vi "parse and execute command.vi"(8 "Python Command":string="scan(0,0,64,64)") -> (1 "Python Return String":string="unknown command:scan\r\n", 2 "exit":bool, 3 "command error":errorcluster)   [LabVIEW 2014]
panel:
  out "Command Folder":path
  out "error out":errorcluster={"status"=TRUE, "code"=7, "source"="Open VI Reference in parse and execute command.vi<APPEND>\nVI Path: <b>D:\\Scripts\\VIs\\SLLServer\\NanonisCommand\\scan.vi</b>"}
  in  "VI Refnum":refnum<vi>
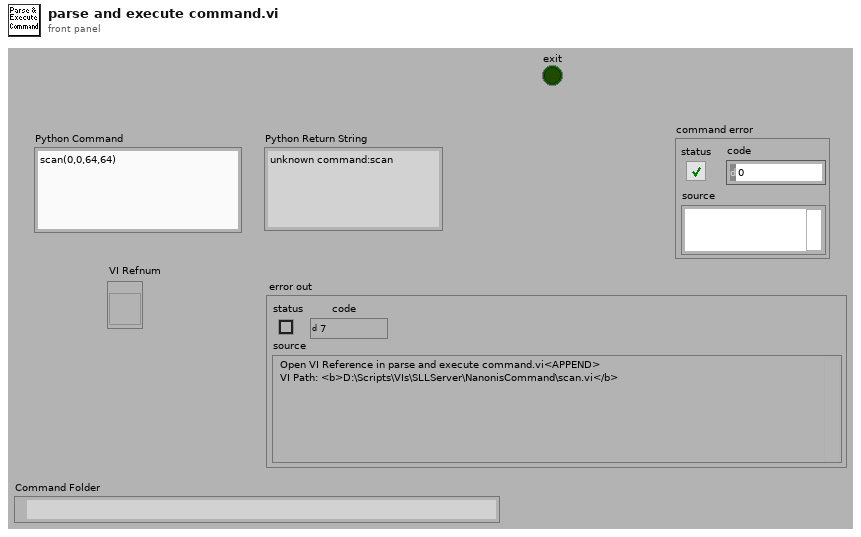
[diagram p1: front panel]
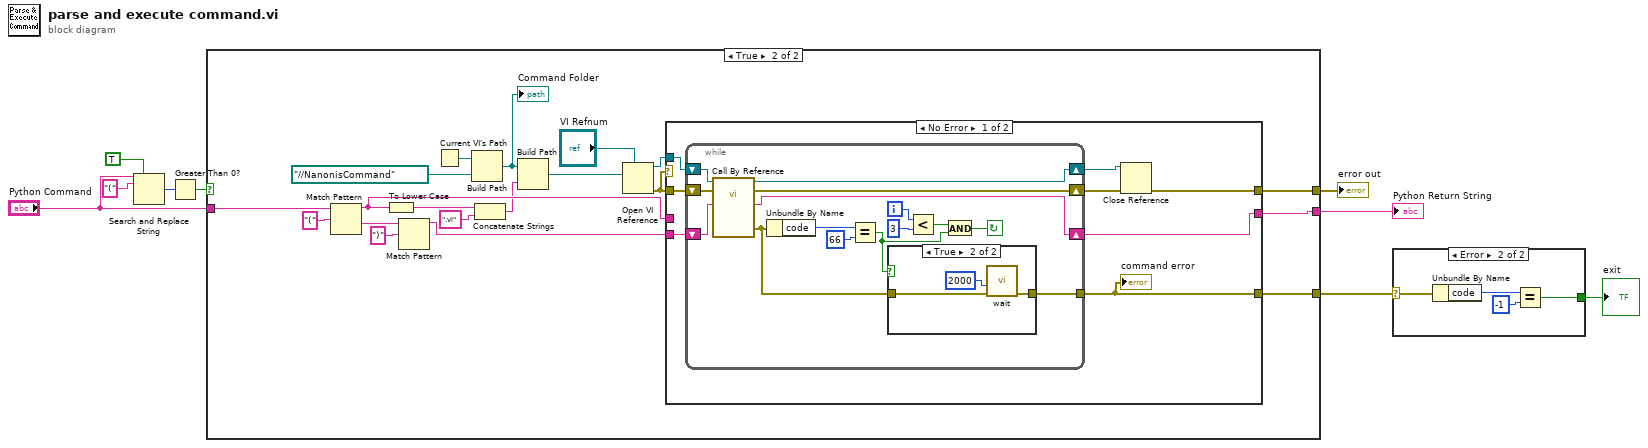
[diagram p0: block diagram]
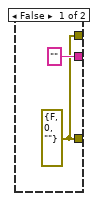
[diagram p2: hidden frame]
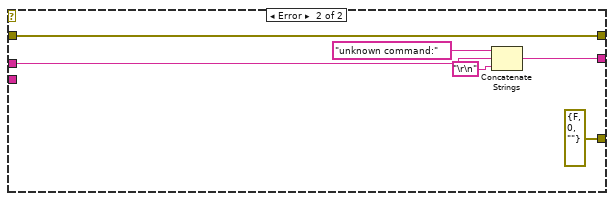
[diagram p4: hidden frame]
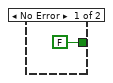
[diagram p5: hidden frame]
diagram:
  n1 = Search and Replace String(replace all?=TRUE ("replace all? (F)"), input string="Python Command", search string="(") -> (number of replacements=w1:i32)  [unwired: 5 in, 3 out]
  n2 = Greater Than 0?(x=w1) -> (x > 0?=w2:bool)
  n3 = case shown="True" w2 {
    tunnel: "Python Command" -> [_ w30]
    tunnel: ["" ("Output") w23] -> w9
    tunnel: [w10 w16] -> w7
    tunnel: [w10 w15] -> w6
    frame False {
      w10 = errorcluster {"status"=FALSE, "code"=0, "source"=""} ("error out")
    }
    frame True {
      n4 = Match Pattern(string=w30, regular expression="(") -> (before substring=w20:string, after substring=w27:string)  [unwired: 1 in, 2 out]
      n5 = To Lower Case(string=w20) -> (all lower case string=w17:string)
      n6 = Match Pattern(string=w27, regular expression=")") -> (before substring=w24:string)  [unwired: 1 in, 3 out]
      n7 = Current VI's Path() -> (path=w13:path)
      n8 = Build Path(base path=w13, name or relative path=path "../../NanonisCommand") -> (appended path=w12:path)
      "Command Folder" <- w12
      n9 = Concatenate Strings(w17, ".vi" ("regular expression")) -> (w18:string)
      n10 = Build Path(base path=w12, name or relative path=w18) -> (appended path=w19:path)
      n11 = Open VI Reference(type specifier VI Refnum (for type only)="VI Refnum", vi path=w19) -> (vi reference=w25:refnum<vi>, error out=w21:errorcluster)  [unwired: 4 in]
      n12 = case shown="No Error" w21 {
        tunnel: w25 -> [w38 _]
        tunnel: w21 -> [w36 w63]
        tunnel: [w34 w63] -> w16
        tunnel: w24 -> [w33 _]
        tunnel: [w32 w59] -> w23
        tunnel: w20 -> [_ w62]
        tunnel: [w31 errorcluster {"status"=FALSE, "code"=0, "source"=""} ("error out")] -> w15
        frame No Error {
          n13 = while {
            tunnel: [w39] -> w31
            shift-right: [w52] -> w37
            shift-left: w38 -> [w53]
            shift-right: [w50] -> w35
            shift-left: w36 -> [w51]
            shift-right: [w48] -> w32
            shift-left: w33 -> [w49]
            i -> [w44]
            stop <- w45 continue-if-true
            n14 = call-by-ref "?"(reference=w53, error in=w51, "Input"=w49) -> (reference out=w52:refnum<vi>, error out=w50:errorcluster, 0:"error out"=w40:errorcluster, "Output"=w48:string)  [unwired: 9 in]
            n15 = Unbundle By Name(w40) -> ("code"=w47:i32)
            n16 = Equal?(x=w47, y=66) -> (x = y?=w41:bool)
            n17 = case shown="True" w41 {
              tunnel: w40 -> [w54 w56]
              tunnel: [w54 w55] -> w39
              frame False {
              }
              frame True {
                n18 = call "wait.vi"("error in"=w56, "milliseconds to wait"=u32 2000) -> ("error out"=w55:errorcluster)  [unwired: 8 in, 1 out]
              }
            }
            n19 = Less?(x=w44, y=3) -> (x < y?=w42:bool)
            n20 = And(x=w42, y=w41) -> (x .and. y?=w45:bool)
          }
          "command error" <- w31
          n21 = Close Reference(reference=w37, error in (no error)=w35) -> (error out=w34:errorcluster)
        }
        frame Error {
          n22 = Concatenate Strings("unknown command:" ("Output"), w62, "\r\n") -> (w59:string)
        }
      }
    }
  }
  "Python Return String" <- w9
  "error out" <- w7
  n23 = case shown="Error" w6 {
    selector: w6 -> [_ w68]
    tunnel: [FALSE w65] -> w8
    frame No Error {
    }
    frame Error {
      n24 = Unbundle By Name(w68) -> ("code"=w67:i32)
      n25 = Equal?(x=w67, y=-1) -> (x = y?=w65:bool)
    }
  }
  "exit" <- w8
